vi "TecellaExample.vi"() -> ()   [LabVIEW 2009]
uses:
  TecellaChannel/TecellaChannel.lvclass
  TecellaClient/TecellaClient.lvclass
panel:
  in  "Samples":dbl=1024.0
  out "Waveform Chart":dbl[][](graph)
  in  "stop":bool
  out "Running?":bool
  out "Is Simulated?":bool
  out "isAlive":bool
  in  "Voltage":dbl
  in  "Channel":i8
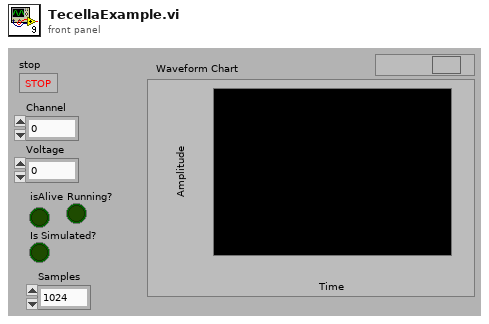
[diagram p1: front panel]
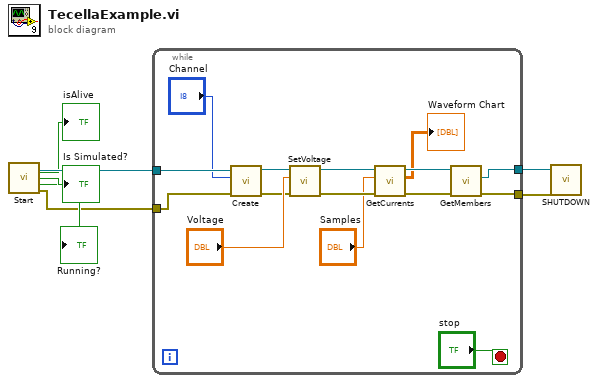
[diagram p0: block diagram]
diagram:
  n1 = call "Start.vi"() -> ("TecellaClient"=w7:refnum<class "TecellaClient.lvclass">, "isAlive"=→"isAlive":bool, "Is Simulated?"=→"Is Simulated?":bool, "Running?"=→"Running?":bool, "error out"=w3:errorcluster)  [unwired: 11 in]
  n2 = while {
    tunnel: w7 -> [w21]
    tunnel: [w8] -> w1
    tunnel: [w16] -> w2
    tunnel: w3 -> [w13]
    stop <- "stop" stop-if-true
    n3 = call "Create.vi"("error in (no error)"=w13, "Channel"="Channel", "TecellaClient.lvclass"=w21) -> ("error out"=w12:errorcluster, "TecellaChannel out"=w20:refnum<class "TecellaChannel.lvclass">)  [unwired: 7 in]
    n4 = call-dynamic "SetVoltage.vi"("error in (no error)"=w12, "Voltage"="Voltage", "TecellaChannel in"=w20) -> ("error out"=w11:errorcluster, "TecellaChannel out"=w19:refnum<class "TecellaChannel.lvclass">)  [unwired: 7 in]
    n5 = call-dynamic "GetCurrents.vi"("error in (no error)"=w11, "Samples"="Samples", "TecellaChannel in"=w19) -> ("error out"=w17:errorcluster, "Currents (nA)"=→"Waveform Chart":dbl[][], "TecellaChannel out"=w18:refnum<class "TecellaChannel.lvclass">)  [unwired: 6 in]
    n6 = call-dynamic "GetMembers.vi"("error in (no error)"=w17, "TecellaChannel in"=w18) -> ("error out"=w16:errorcluster, "TecellaClient.lvclass"=w8:refnum<class "TecellaClient.lvclass">)  [unwired: 6 in, 2 out]
  }
  n7 = call-dynamic "SHUTDOWN.vi"("error in (no error)"=w2, "TecellaClient in"=w1) -> ()  [unwired: 8 in, 2 out]
